vi "ProcessName.vi"() -> (1 "process name":string)   [LabVIEW 2017, in "IrAcquisition.lvlib"]
uses:
  <vilib>/addons/InsightCM/Devices/Shared/Ir/IrAcquisition/IrAcquisition.lvlib
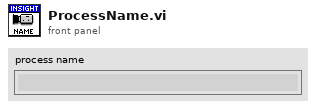
[diagram p1: front panel]
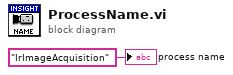
[diagram p0: block diagram]
diagram:
  "process name" <- "IrImageAcquisition" ("ProcessName")
